vi "set keyswitch state.vi"(8 "error in (no error)":errorcluster, 11 "Cobolt in":refnum<class "Cobolt.lvclass">) -> (0 "error out":errorcluster, 3 "Cobolt out":refnum<class "Cobolt.lvclass">)   [LabVIEW 2012, in "Cobolt.lvclass"]
uses:
  Cobolt.lvclass
  CoboltLaserDrivers_Public_LV2012/CoboltLaser_Controls/ExpectedResponseType.ctl
  Cobolt.lvclass/Cobolt.ctl
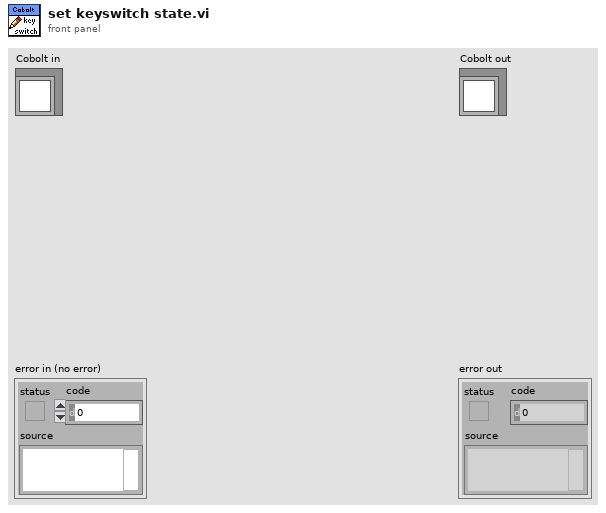
[diagram p1: front panel]
types:
  T1 = typedef "Cobolt.lvclass/ExpectedResponseType.ctl" = u16
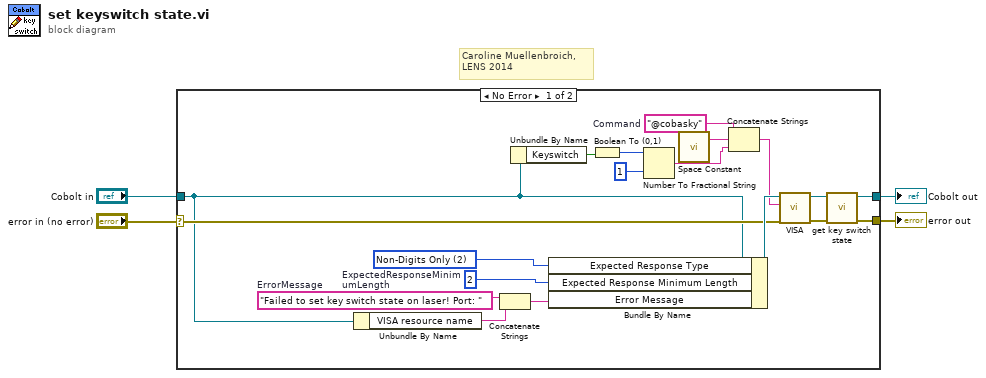
[diagram p0: block diagram]
diagram:
  # "Caroline Muellenbroich, \nLENS 2014"
  n1 = case shown="No Error" "error in (no error)" {
    selector: "error in (no error)" -> [w15 w25]
    tunnel: [w9 w25] -> w3
    tunnel: [w7 w24] -> w1
    tunnel: "Cobolt in" -> [w12 w24]
    frame No Error {
      w23 = T1 2 items=["Any", "Digits Only", "Non-Digits Only"] ("ExpectedResponseType")
      w19 = 2  # ExpectedResponseMinimumLength
      w21 = "Failed to set key switch state on laser! Port: "  # ErrorMessage
      w16 = "@cobasky"  # Command
      n2 = Unbundle By Name(w12) -> ("VISA resource name"=w20:string)
      n3 = Concatenate Strings(w21, w20) -> (w22:string)
      n4 = Unbundle By Name(w12) -> ("Keyswitch"=w11:bool)
      n5 = Bundle By Name(cluster=w12, "Expected Response Type"=w23, "Expected Response Minimum Length"=w19, "Error Message"=w22) -> (w18:refnum<class "Cobolt.lvclass">)
      n6 = Boolean To (0,1)(Boolean=w11) -> (0, 1=w13:i16)
      n7 = Number To Fractional String(number=w13, precision (6)=i16 1) -> (F-format string=w6:string)  [unwired: 2 in]
      n8 = call <vilib>:"Space Constant.vi"() -> ("String"=w5:string)
      n9 = Concatenate Strings(w16, w5, w6) -> (w17:string)
      n10 = call-dynamic "VISA.vi"("error in (no error)"=w15, "string to write"=w17, "Cobolt in"=w18) -> ("error out"=w10:errorcluster, "Cobolt out"=w8:refnum<class "Cobolt.lvclass">)  [unwired: 6 in, 1 out]
      n11 = call-dynamic "get key switch state.vi"("error in (no error)"=w10, "Cobolt in"=w8) -> ("error out"=w9:errorcluster, "Cobolt out"=w7:refnum<class "Cobolt.lvclass">)  [unwired: 8 in]
    }
    frame Error {
    }
  }
  "error out" <- w3
  "Cobolt out" <- w1
